vi "mt.vi"(6 "数值":dbl, 9 "布尔":bool, 10 "名称或相对路径":path, 11 "基路径":path) -> (3 "数组":string[][](array[string]))   [LabVIEW 2022 SP3]
uses:
  <vilib>/Utility/file.llb/Write Delimited Spreadsheet (string).vi
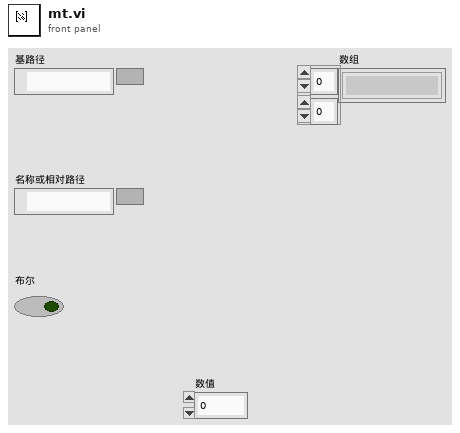
[diagram p1: front panel]
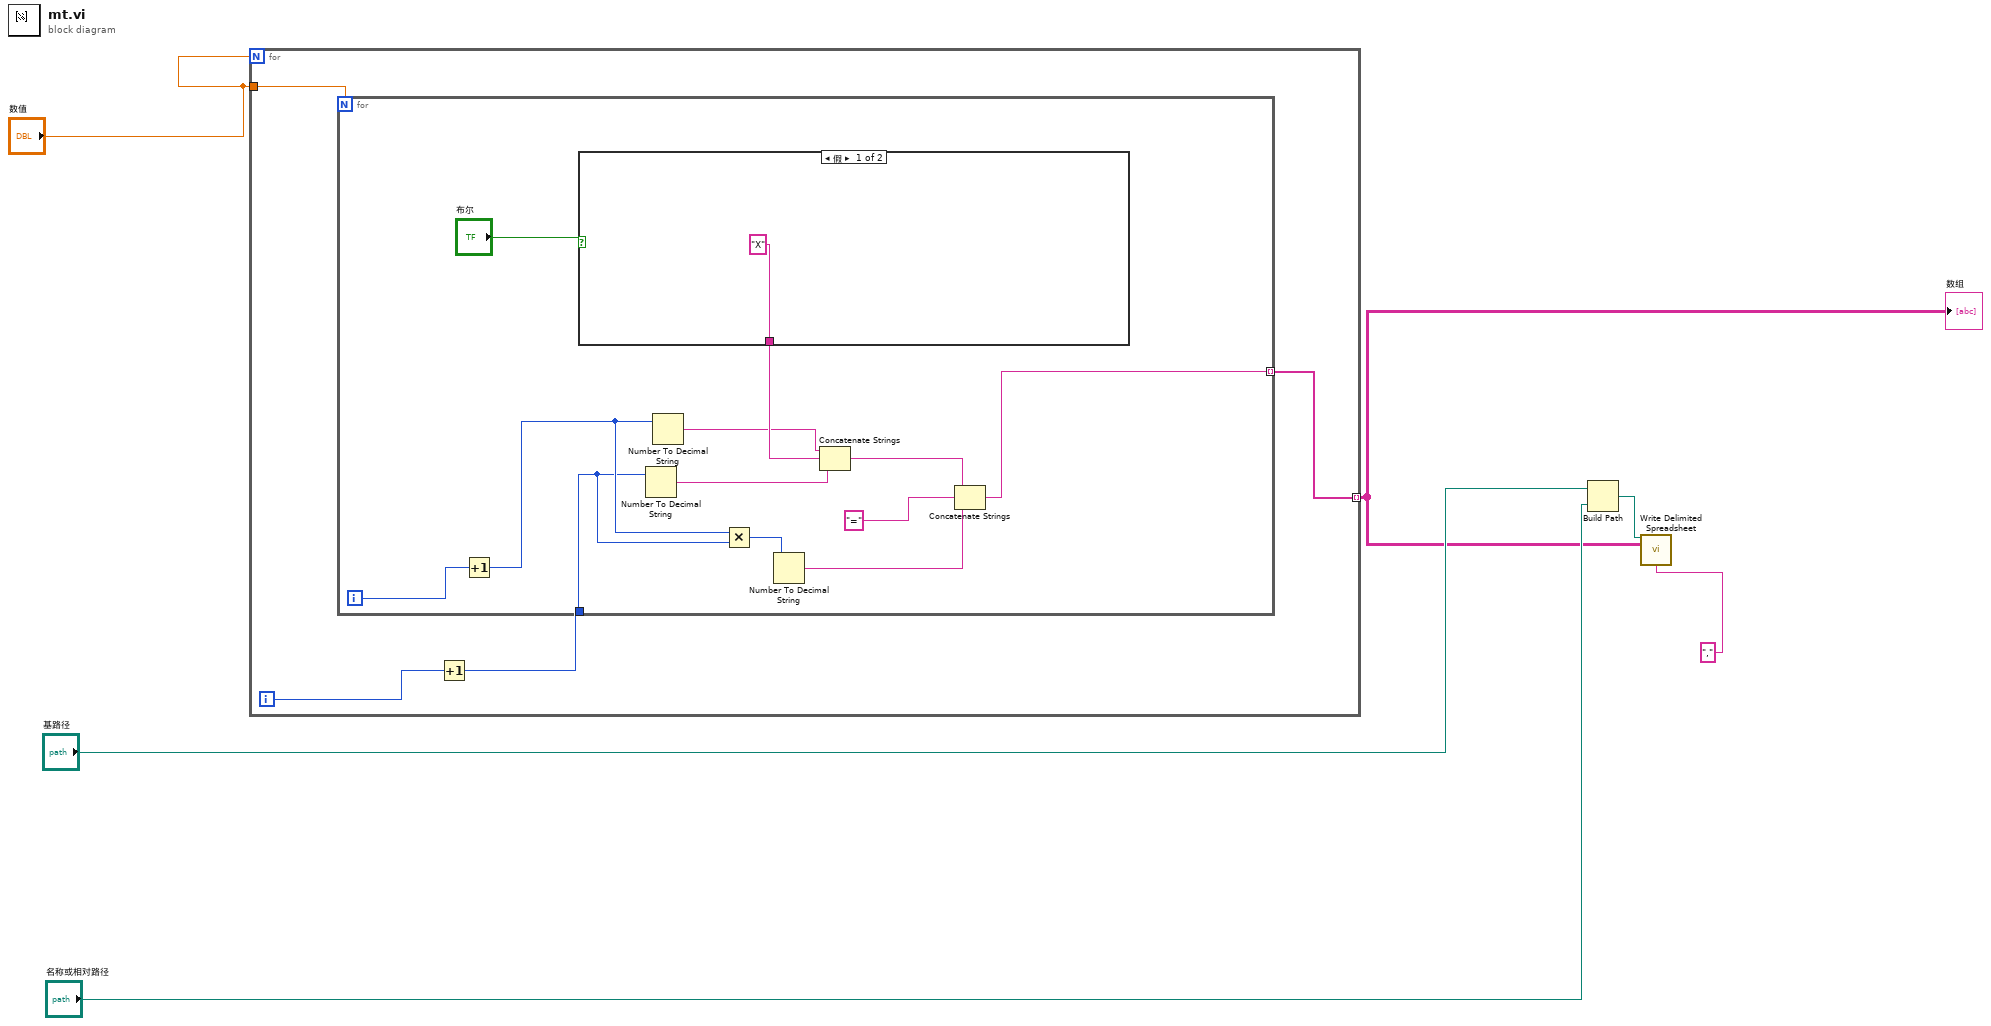
[diagram p0: block diagram]
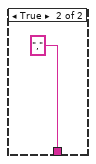
[diagram p2: hidden frame]
diagram:
  n1 = for {
    N: "数值" -> [_]
    tunnel: "数值" -> [w10]
    tunnel: [w7] -> w2 mode=indexing
    i -> [w9]
    n2 = Increment(x=w9) -> (x+1=w8:i32)
    n3 = for {
      N: w10 -> [_]
      tunnel: w8 -> [w19]
      tunnel: [w11] -> w7 mode=indexing
      i -> [w21]
      n4 = Increment(x=w21) -> (x+1=w20:i32)
      n5 = case shown="假" "布尔" {
        tunnel: ["X" ","] -> w18
        frame False {
        }
        frame True {
        }
      }
      n6 = Number To Decimal String(number=w19) -> (decimal integer string=w16:string)  [unwired: 1 in]
      n7 = Number To Decimal String(number=w20) -> (decimal integer string=w17:string)  [unwired: 1 in]
      n8 = Multiply(x=w20, y=w19) -> (x*y=w13:i32)
      n9 = Number To Decimal String(number=w13) -> (decimal integer string=w12:string)  [unwired: 1 in]
      n10 = Concatenate Strings(w17, w18, w16) -> (w14:string)
      n11 = Concatenate Strings(w14, "=" ("字符串"), w12) -> (w11:string)
    }
  }
  "数组" <- w2
  n12 = Build Path(base path="基路径", name or relative path="名称或相对路径") -> (appended path=w3:path)
  n13 = call-poly <vilib>:"Write Delimited Spreadsheet.vi"("file path (dialog if empty)"=w3, "2D data"=w2, "delimiter (\\t)"="," ("delimiter (\\t)")) -> ()  [unwired: 11 in, 2 out]
